vi "st_Neg Binomial PDF (kx).vi"(9 "p":dbl=0.5, 10 "x":dbl=5.0, 11 "ky":dbl) -> (0 "error":i32, 3 "pdf(ky)":dbl=0.03125)   [LabVIEW 2024, in "NI_Gmath.lvlib"]
uses:
  NI_Gmath.lvlib
  st_error_code.ctl
panel:
  # "Negative Binomial PDF(ky)"
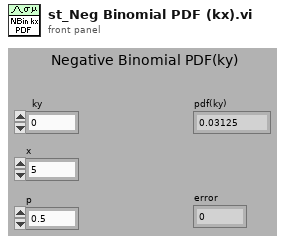
[diagram p1: front panel]
types:
  T1 = typedef "NI_Gmath.lvlib/st_error_code.ctl" = i32
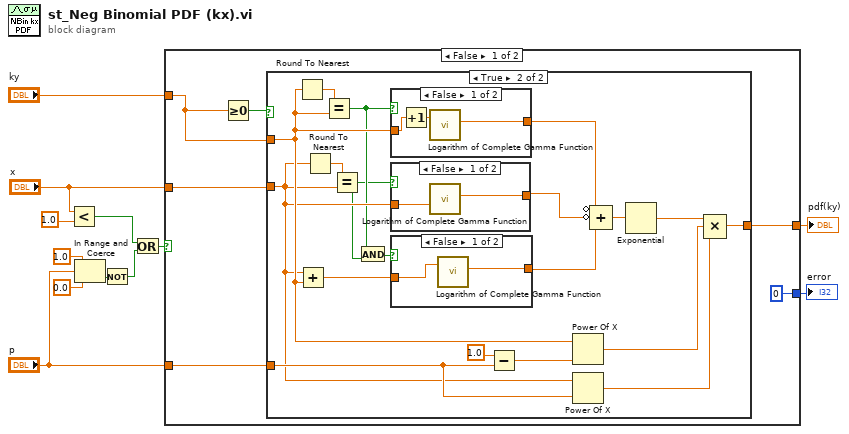
[diagram p0: block diagram]
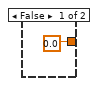
[diagram p2: hidden frame]
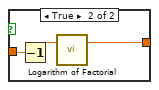
[diagram p3: hidden frame]
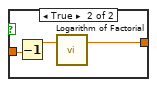
[diagram p4: hidden frame]
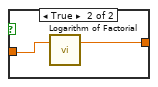
[diagram p5: hidden frame]
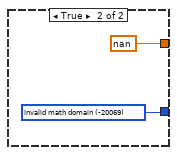
[diagram p6: hidden frame]
diagram:
  n1 = Less?(x="x", y=1.0) -> (x < y?=w2:bool)
  n2 = In Range and Coerce(upper limit=1.0, x="p", lower limit=0.0) -> (In Range?=w4:bool)  [unwired: 1 out]
  n3 = Not(x=w4) -> (.not. x?=w3:bool)
  n4 = Or(x=w2, y=w3) -> (x .or. y?=w7:bool)
  n5 = case shown="False" w7 {
    tunnel: [0 ("invalid math domain") w54] -> w12
    tunnel: [w15 nan] -> w11
    tunnel: "ky" -> [w14 _]
    tunnel: "x" -> [w17 _]
    tunnel: "p" -> [w16 _]
    frame False {
      n6 = Greater Or Equal To 0?(x=w14) -> (x >= 0?=w13:bool)
      n7 = case shown="True" w13 {
        tunnel: [0.0 w33] -> w15
        tunnel: w14 -> [_ w30]
        tunnel: w17 -> [_ w27]
        tunnel: w16 -> [_ w37]
        frame False {
        }
        frame True {
          n8 = Round To Nearest(number=w30) -> (nearest integer value=w31:dbl)
          n9 = Add(x=w27, y=w30) -> (x+y=w20:dbl)
          n10 = Round To Nearest(number=w27) -> (nearest integer value=w28:dbl)
          n11 = Equal?(x=w31, y=w30) -> (x = y?=w26:bool)
          n12 = Equal?(x=w28, y=w27) -> (x = y?=w25:bool)
          n13 = And(x=w26, y=w25) -> (x .and. y?=w24:bool)
          n14 = case shown="False" w26 {
            tunnel: w30 -> [w50 w53]
            tunnel: [w49 w52] -> w21
            frame False {
              n15 = Increment(x=w50) -> (x+1=w51:dbl)
              n16 = call "Logarithm of Complete Gamma Function.vi"("x"=w51) -> ("ln(g(x))"=w49:dbl)  [unwired: 2 in]
            }
            frame True {
              n17 = call "Logarithm of Factorial.vi"("n"=w53) -> ("ln(n!)"=w52:dbl)  [unwired: 2 in]
            }
          }
          n18 = case shown="False" w25 {
            tunnel: w27 -> [w44 w48]
            tunnel: [w45 w47] -> w23
            frame False {
              n19 = call "Logarithm of Complete Gamma Function.vi"("x"=w44) -> ("ln(g(x))"=w45:dbl)  [unwired: 2 in]
            }
            frame True {
              n20 = Decrement(x=w48) -> (x-1=w46:dbl)
              n21 = call "Logarithm of Factorial.vi"("n"=w46) -> ("ln(n!)"=w47:dbl)  [unwired: 2 in]
            }
          }
          n22 = case shown="False" w24 {
            tunnel: w20 -> [w39 w43]
            tunnel: [w40 w42] -> w22
            frame False {
              n23 = call "Logarithm of Complete Gamma Function.vi"("x"=w39) -> ("ln(g(x))"=w40:dbl)  [unwired: 2 in]
            }
            frame True {
              n24 = Decrement(x=w43) -> (x-1=w41:dbl)
              n25 = call "Logarithm of Factorial.vi"("n"=w41) -> ("ln(n!)"=w42:dbl)  [unwired: 2 in]
            }
          }
          n26 = Subtract(x=1.0 ("t"), y=w37) -> (x-y=w38:dbl)
          n27 = Power Of X(1:w38, 2:w30) -> (0:w35:dbl)
          n28 = Power Of X(1:w37, 2:w27) -> (0:w34:dbl)
          n29 = Compound Arithmetic op=ADD(invert w21, invert w23, w22) -> (w29:dbl)
          n30 = Exponential(1:w29) -> (0:w32:dbl)
          n31 = Compound Arithmetic op=MULTIPLY(w32, w35, w34) -> (w33:dbl)
        }
      }
    }
    frame True {
      w54 = T1 -20069 items=["invalid math domain"=-20069, "Fourier interpolation size m >= n"=-20070, "empty array"=-20003] ("stat interp error code")
    }
  }
  "pdf(ky)" <- w11
  "error" <- w12
